vi "WPI_RobotDriveHolonomicDrive.vi"   [LabVIEW 2017]
doc: "Configures the motors for holonomic driving. Holonomic driving allows you to move the robot in any direction without first rotating or maneuvering the robot. Use the Selector to choose an appropriate control method for your robot's drive.\n\nThis software is licensed. Open the labview\\readme\\WPI Robotics Library Open Source License.txt file for more information."
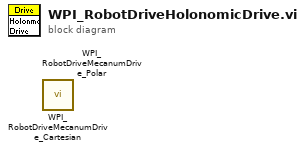
[diagram p0: block diagram]
diagram:
  n1 = call <vilib>:"WPI_RobotDriveMecanumDrive_Cartesian.vi"() -> ()  [unwired: 9 in, 3 out]
  n2 = call <vilib>:"WPI_RobotDriveMecanumDrive_Polar.vi"() -> ()  [unwired: 9 in, 3 out]
